vi "Read Config FIFO.vi"(8 "error in (no error)":errorcluster, 11 "RT Data in":T1 {"Label Transfer Config"."Block Data Refs"."Data Reference" format="%.0x"; "Status Config"."HWOut Dur Ref" format="%.0x"; "Status Config"."HWIn Dur Ref" format="%.0x"; "Status Config"."Error Data Ref" format="%.0x"; "HWOutput Channels"."Labels Settings"."Label" format="%.0o"; "HWInput Channels"."Labels Settings"."Label" format="%.0o"}) -> (0 "error out":errorcluster, 3 "RT Data out":T1 {"Label Transfer Config"."Block Data Refs"."Data Reference" format="%.0x"; "Status Config"."HWOut Dur Ref" format="%.0x"; "Status Config"."HWIn Dur Ref" format="%.0x"; "Status Config"."Error Data Ref" format="%.0x"; "HWOutput Channels"."Labels Settings"."Label" format="%.0o"; "HWInput Channels"."Labels Settings"."Label" format="%.0o"})   [LabVIEW 2012, in "AIT 429 Engine.lvlib"]
uses:
  AIT 429 Engine.lvlib
  RT Controls/RT Data.ctl
  RT Controls/RT HW Channel.ctl
  RT Controls/RT Label Settings.ctl
  Shared/Controls and Global/Label.ctl
  Shared/Controls and Global/transferPeriod.ctl
  RT Controls/Driver Data.ctl
  RT Controls/RT Word Settings.ctl
  <vilib>/NI Veristand/Custom Device API/Block Data Reference.ctl
  <vilib>/NI Veristand/Custom Device API/Data Reference.ctl
  RT Controls/RT Param Setting.ctl
  Shared/Controls and Global/Start Bit.ctl
  Shared/Controls and Global/Number of Bits.ctl
  Shared/Controls and Global/TransferType.ctl
  RT Controls/Error Qs.ctl
  RT Controls/Status Channels Config.ctl
  RT Controls/FIFO.ctl
  RT Controls/Label Transfer Config.ctl
  ARINC 429 Shared.lvlib
  <vilib>/NI Veristand/Custom Device API/Custom Device API.lvlib
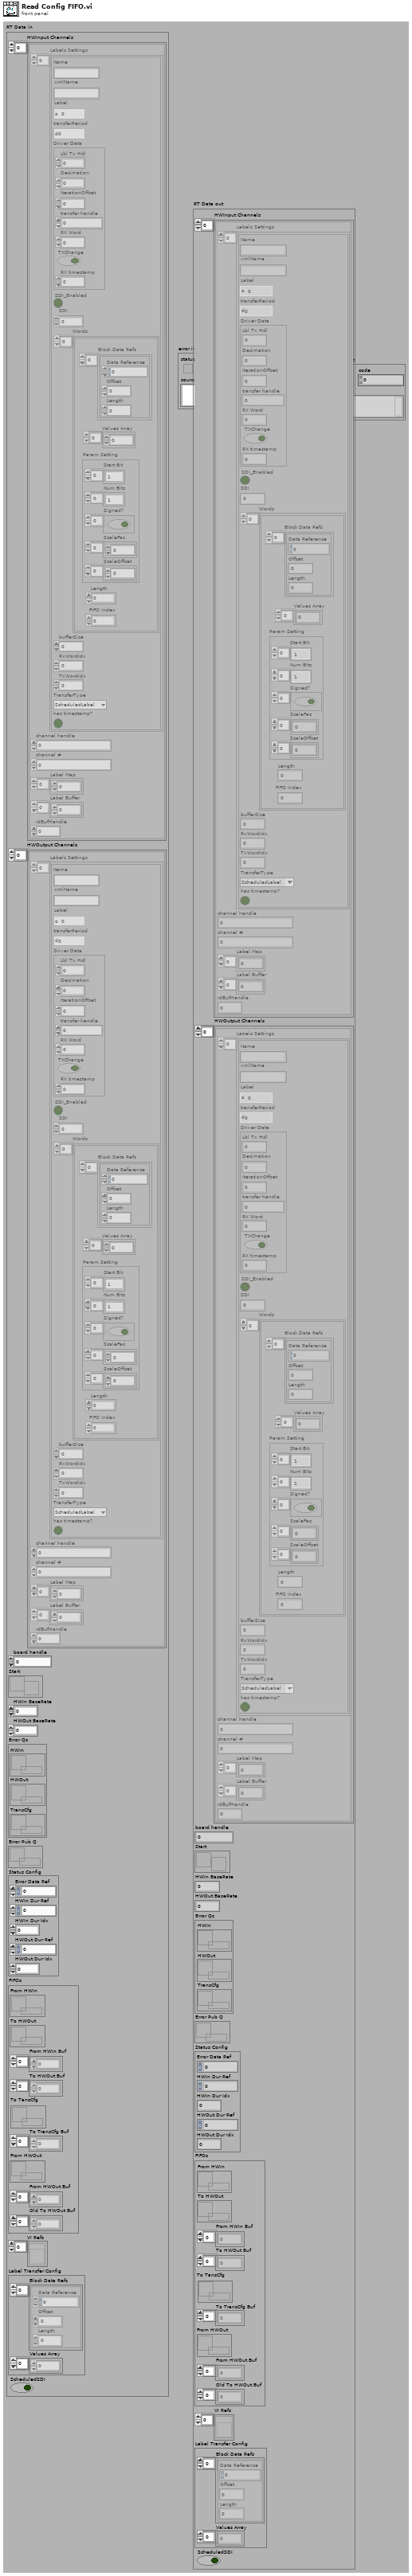
[diagram p1: front panel]
types:
  T1 = typedef "AIT 429 Engine.lvlib/RT Data.ctl" = cluster{"HWInput Channels":T2[], "HWOutput Channels":T2[], "board handle":u32, "Start":refnum<notifier>, "HWIn BaseRate":i64, "HWOut BaseRate":i64, "Error Qs":T14, "Error Pub Q":refnum<queue>, "Status Config":T15, "FIFOs":T16, "VI Refs":refnum<vi>[], "Label Transfer Config":T17, "ScheduledSDI":bool}
  T2 = typedef "AIT 429 Engine.lvlib/RT HW Channel.ctl" = cluster{"Labels Settings":T3[], "channel handle":u32, "channel #":u16, "Label Map":i32[], "Label Buffer":u32[], "rdBufHandle":u32}
  T3 = typedef "AIT 429 Engine.lvlib/RT Label Settings.ctl" = cluster{"Name":string, "xmlName":string, "Label":T4, "transferPeriod":T5, "Driver Data":T6, "SDI_Enabled":bool, "SDI":u8, "Words":T7[], "bufferSize":u32, "RxWordIdx":i32, "TxWordIdx":i32, "TransferType":T13, "has timestamp?":bool}
  T4 = typedef "ARINC 429 Shared.lvlib/Label.ctl" = u8
  T5 = typedef "ARINC 429 Shared.lvlib/transferPeriod.ctl" = u32
  T6 = typedef "AIT 429 Engine.lvlib/Driver Data.ctl" = cluster{"Lbl Tx Hdl":u32, "Decimation":i32, "IterationOffset":i32, "transfer handle":u32, "RX Word":u32, "TXChange":bool, "RX timestamp":dbl}
  T7 = typedef "AIT 429 Engine.lvlib/RT Word Settings.ctl" = cluster{"Block Data Refs":T8[], "Values Array":dbl[], "Length":i32, "FIFO Index":i32, "Param Setting":T10}
  T8 = typedef "Custom Device API.lvlib/Block Data Reference.ctl" = cluster{"Data Reference":T9, "Offset":i32, "Length":i32}
  T9 = typedef "Custom Device API.lvlib/Data Reference.ctl" = i32
  T10 = typedef "AIT 429 Engine.lvlib/RT Param Setting.ctl" = cluster{"Start Bit":T11[], "Num Bits":T12[], "Signed?":bool[], "ScaleFac":dbl[], "ScaleOffset":dbl[]}
  T11 = typedef "ARINC 429 Shared.lvlib/Start Bit.ctl" = i32
  T12 = typedef "ARINC 429 Shared.lvlib/Number of Bits.ctl" = i32
  T13 = typedef "ARINC 429 Shared.lvlib/TransferType.ctl" = enum16{"ScheduledLabel", "Acyclic", "Block", "Strobe"}
  T14 = typedef "AIT 429 Engine.lvlib/Error Qs.ctl" = cluster{"HWIn":refnum<queue>, "HWOut":refnum<queue>, "TransCfg":refnum<queue>}
  T15 = typedef "AIT 429 Engine.lvlib/Status Channels Config.ctl" = cluster{"Error Data Ref":T9, "HWIn Dur Ref":T9, "HWIn Dur Idx":i32, "HWOut Dur Ref":T9, "HWOut Dur Idx":i32}
  T16 = typedef "AIT 429 Engine.lvlib/FIFO.ctl" = cluster{"From HWIn":refnum<k33>, "To HWOut":refnum<k33>, "From HWIn Buf":dbl[], "To HWOut Buf":dbl[], "To TansCfg":refnum<k33>, "To TransCfg Buf":dbl[], "From HWOut":refnum<k33>, "From HWOut Buf":dbl[], "Old To HWOut Buf":dbl[]}
  T17 = typedef "AIT 429 Engine.lvlib/Label Transfer Config.ctl" = cluster{"Block Data Refs":T8[], "Values Array":dbl[]}
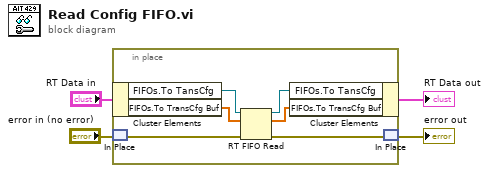
[diagram p0: block diagram]
diagram:
  n1 = in-place {
    n2 = in-place-cluster #1("RT Data in") -> ("FIFOs.To TansCfg"=w10:refnum<k33>, "FIFOs.To TransCfg Buf"=w9:dbl[])
    n3 = in-place-match #2("error in (no error)") -> (w6:errorcluster)
    n4 = RT FIFO Read(0:w10, 1:w9, 3:w6) -> (8:w7:refnum<k33>, 9:w8:dbl[], 11:w5:errorcluster)  [unwired: 1 in, 2 out]
    n5 = in-place-cluster #1("FIFOs.To TansCfg"=w7, "FIFOs.To TransCfg Buf"=w8) -> (→"RT Data out":T1)
    n6 = in-place-match #2(w5) -> (→"error out":errorcluster)
  }
